vi "MarvinReport.vi"(0 "HEADER1":string="===================================================================\r\n||  Functional and Performance Test  For  DUAL-SERVO- L O W E R  ||\r\n||  P/N  TLM132XX501    S/N:001    Power-Input:18,28,32 +/-0.5V  ||\r\n||  Date:6/12/2007    Time: 15-00  Test-Conductor: Itzik         ||\r\n||  Tester P/N yyyy-yyyyyy-yyyy    S/N:01                        ||\r\n||  POWER SUPPLY P/N xxxxx                                       ||\r\n||  Remarks:                                                     ||\r\n||  You can write here what ever you want                        ||\r\n||                                                               ||\r\n===================================================================", 1 "ATR Or":refnum<vi>, 2 "Steps   pfull":string[][](table)=array602x15[9030 elements] caption="ATR", 3 "Footer UUT":string, 5 "pageNum":i32=13, 6 "InputHeaderArray":string[][](array[string]), 7 "FILE NAME":string="d", 9 "Report Folder":path=path "C:/EPD/ATRS", 11 "PN":string, 12 "error in (no error)":errorcluster, 13 "REV":string, 14 "Test-Conductor":string) -> (4 "path out":path, 15 "error out":errorcluster)   [LabVIEW 2017]
uses:
  <vilib>/Utility/miscctls.llb/LVRowAndColumnUnsignedTypeDef.ctl
  <vilib>/Utility/NIReport.llb/Append Image to Report (path wrap).vi
  <vilib>/Utility/NIReport.llb/Append Text Table to Report (wrap).vi
  <vilib>/Utility/NIReport.llb/Append Report Text (str wrap).vi
  <vilib>/Utility/NIReport.llb/NI_report.lvclass
  <vilib>/Utility/NIReport.llb/Word/NI_Word.lvclass
  <vilib>/addons/_office/NI_ReportGenerationToolkit.lvlib
panel:
  out "Steps   p31":string[][](table)=[["6.1", "Visual Inspection", "", "", "", "", ""], ["6.1.1", "Verification of Components Not Installed", "N/A", "-", "", "", ""], ["", "", "", "", "", "", ""], ["6.1.2", "Manufacturing Defects", "N/A", "-", "", "", ""], ["", "", "", "", "", "", ""], ["6.2", "Power Supply Testing", "", "", "", "", ""], ["6.2.1", "Input Current Drawn", "", "", "", "", ""], ["6.2.1.1", "DC Input Current", "< 150", "-", "mA", "", ""], ["", "", "", "", "", "", ""], ["6.2.2", "Power Supply Voltages", "", "", "", "", ""], ["6.2.2.1", "12V", "12.0", "+/-0.500", "V", "", ""], ["6.2.2.2", "5V", "5.0", "+/-0.200", "V", "", ""], ["6.2.2.3", "3.3V", "3.3", "+/-0.100", "V", "", ""], ["6.2.2.4", "1.8V", "1.8", "+/-0.100", "V", "", ""], ["", "", "", "", "", "", ""], ["7", "Functional Test Procedure", "", "", "", "", ""], ["7.1", "Weight Check", "4180", "+/-10.00", "gr", "", ""], ["", "", "", "", "", "", ""], ["7.2", "Insulation Resistance Test", "", "", "", "", ""], ["7.2.1", "J3.B to Chassis", "> 1M", "-", "ohms", "", ""], ["7.2.2", "J1.16 to Chassis", "> 100K", "-", "ohms", "", ""], ["", "", "", "", "", "", ""], ["7.2", "Bonding Resistance", "", "", "", "", ""], ["7.2.3", "J1 Body to Chassis", "< 2m", "-", "ohms", "", ""], ["7.2.4", "J2  Body to Chassis", "< 2m", "-", "ohms", "", ""], ["7.2.5", "J3  Body to Chassis", "< 2m", "-", "ohms", "", ""], ["", "", "", "", "", "", ""], ["7.2.1", "CANbus Resistance Test", "", "", "", "", ""], ["7.2.1.1", "J1.17 to J1.18", "> 10K", "-", "ohms", "", ""], ["", "", "", "", "", "", ""], ["7.3", "Sealing Test", "N/A", "-", "", "", ""], ["", "", "", "", "", "", ""], ["7.4", "Communication Test", "", "", "", "", ""], ["7.4.1", "Serial RS-232", "N/A", "-", "", "", ""], ["7.4.2", "CAN Bus", "N/A", "-", "", "", ""], ["", "", "", "", "", "", ""], ["7.5", "Performances Tests", "", "", "", "", ""], ["7.5.1", "Reverse Polarity Test", "", "", "", "", ""], ["7.5.1.1", "DC Input Current", "< 1", "-", "mA", "", ""], ["", "", "", "", "", "", ""], ["7.5.2", "Enable Test", "", "", "", "", ""], ["7.5.2.1", "Fan Speed before Opened Enable ", "6000", "+/-200.0", "rpm", "", ""], ["7.5.2.2", "Fan Speed at Opened Enable ", "0", "+/-200.0", "rpm", "", ""], ["7.5.2.3", "Fan Speed at Closed Enable ", "6000", "+/-200.0", "rpm", "", ""], ["7.5.2.4", "Motor Rotation Direction", "Counter-clockwise (Inlet)", "-", "", "", ""], ["", "", "", "", "", "", ""], ["7.5.3", "Stop Time Test ", "", "", "", "", ""], ["7.5.3.1", "Motor Stop time", "< 50", "-", "sec", "", ""], ["", "", "", "", "", "", ""], ["7.5.4", "Speed Command Test", "", "", "", "", ""], ["7.5.4.1", "Fan Speed", "6000", "+/-200.0", "rpm", "", ""], ["7.5.4.2", "Fan Speed", "11500", "+/-200.0", "rpm", "", ""], ["7.5.4.3", "Fan Speed", "15100", "+/-200.0", "rpm", "", ""], ["", "", "", "", "", "", ""], ["7.5.5", "Temperature Sensor Calibration Test", "", "", "", "", ""], ["7.5.5.1", "Sensor Reading Analog Offset", "0", "+/-0.100", ".", "", ""], ["", "", "", "", "", "", ""], ["7.5.6", "Temperature Control Algorithm Test", "", "", "", "", ""], ["7.5.6.1", "Tair <   68 ± 2 oC", "6000", "+/-200.0", "rpm", "", ""], ["7.5.6.2", "Measured Temp.", "", "", "Deg.", "", ""], ["7.5.6.3", "Tair >= 68 ± 2 oC", "11500", "+/-200.0", "rpm", "", ""], ["7.5.6.4", "Transition Temp.", "", "", "Deg.", "", ""], ["7.5.6.5", "Tair >= 88 ± 2 oC", "15100", "+/-400.0", "rpm", "", ""], ["7.5.6.6", "Transition Temp.", "", "", "Deg.", "", ""], ["7.5.6.7", "Tair <= 80 ± 2 oC", "11500", "+/-200.0", "rpm", "", ""], ["7.5.6.8", "Transition Temp.", "", "", "Deg.", "", ""], ["7.5.6.9", "Tair <= 60 ± 2 oC", "6000", "+/-200.0", "rpm", "", ""], ["7.5.6.10", "Transition Temp.", "", "", "Deg.", "", ""], ["", "", "", "", "", "", ""], ["7.5.7", "Burn-in Test", "", "", "", "", ""], ["7.5.7.1", "DC Input Current", "50", "+/-7.000", "A", "", ""], ["7.5.7.2", "Fan Speed", "15100", "+/-400.0", "rpm", "", ""], ["7.5.7.3", "Ambient Temperature", "25", "+/-13.00", "Deg.", "", ""], ["7.5.7.4", "After 10 min of operation", "", "-", "Deg.", "", ""], ["7.5.7.5", "After 20 min of operation", "", "-", "Deg.", "", ""], ["7.5.7.6", "After 30 min of operation", "", "-", "Deg.", "", ""], ["", "", "", "", "", "", ""], ["8", "Auxiliary", "", "", "", "", ""], ["8.1", "Auxiliary Cooling Fan ON", "60", "+/-2.00", "Deg.", "", ""], ["8.2", "Fan status", "ON", "-", "-", "", ""], ["8.3", "Auxiliary Cooling Fan OFF", "55", "+/-2.00", "Deg.", "", ""], ["8.4", "Fan status", "OFF", "-", "-", "", ""], ["", "", "", "", "", "", ""], ["9", "Motor Temp. Test", "", "", "", "", ""], ["9.1", "60 Degree", "60", "+/-2.00", "Deg.", "", ""], ["9.2", "90 Degree", "90", "+/-2.00", "Deg.", "", ""], ["9.3", "110 Degree", "110", "+/-2.00", "Deg.", "", ""]] caption="ATR"
  out "error out 2":errorcluster
  out "RefArr":u32[](array[numeric])
  in  "Tab Control":T1(tab)=enum."Headers and more"
  out "ERRORS\nLIST":string="<pre>Summery of Results (Fails Only) :   Pos.Cmnd.=0.5V F.B. - FAIL !\t   \nPos.Cmnd.=2.0V F.B. - FAIL !\t       Pos.Cmnd.=4.5V F.B. - FAIL !\t  \nPos.Cmnd.=0.5V F.B  - FAIL !\t       Pos.Cmnd.=2.0V F.B. - FAIL !\t\nPos.Cmnd.=4.5V F.B. - FAIL !\t       Pot. / Pos.Cmnd. 1.5v - FAIL !\t   \nPot./Pos.Cmnd.2.0v  - FAIL !\t       Pot. / Pos.Cmnd. 3.5v - FAIL !\t   \nRelay-->RESET  - FAIL !\t            Relay --> SET - FAIL !\t</pre>"
  out "Steps   p1":string[][](table)=[["Load Firmware - reset", "-", "-", "-", "-", ""], ["Test Communication", "-", "-", "-", "-", ""], ["Set S/N", "-", "-", "-", "-", ""], ["Set Board Number", "-", "-", "-", "-", ""], [" ", "", "", "", "", ""], ["Test Communication", "-", "-", "-", "-", ""], ["Get S/N", "-", "-", "-", "", ""], ["Get Board Number", "-", "-", "-", "", ""], ["Get FW", "-", "-", "-", "", ""], ["Small position command", "", "", "", "", ""], ["Measure delta", "", "", "", "", ""], ["Velocity command", "", "", "", "", ""], ["Velocity command", "", "", "", "", ""], ["Velocity command", "", "", "", "", ""], ["Velocity command", "", "", "", "", ""], ["Velocity command", "", "", "", "", ""]] caption="ATR"
  out "Steps   p2":string[][](table)=[["Load Firmware - reset", "-", "-", "-", "-", ""], ["Test Communication", "-", "-", "-", "-", ""], ["Set S/N", "-", "-", "-", "-", ""], ["Set Board Number", "-", "-", "-", "-", ""], [" ", "", "", "", "", ""], ["Test Communication", "-", "-", "-", "-", ""], ["Get S/N", "-", "-", "-", "", ""], ["Get Board Number", "-", "-", "-", "", ""], ["Get FW", "-", "-", "-", "", ""], ["Small position command", "", "", "", "", ""], ["Measure delta", "", "", "", "", ""], ["Velocity command", "", "", "", "", ""], ["Velocity command", "", "", "", "", ""], ["Velocity command", "", "", "", "", ""], ["Velocity command", "", "", "", "", ""], ["Velocity command", "", "", "", "", ""]] caption="ATR"
  out "Steps   p3":string[][](table)=[["Load Firmware - reset", "-", "-", "-", "-", ""], ["Test Communication", "-", "-", "-", "-", ""], ["Set S/N", "-", "-", "-", "-", ""], ["Set Board Number", "-", "-", "-", "-", ""], [" ", "", "", "", "", ""], ["Test Communication", "-", "-", "-", "-", ""], ["Get S/N", "-", "-", "-", "", ""], ["Get Board Number", "-", "-", "-", "", ""], ["Get FW", "-", "-", "-", "", ""], ["Small position command", "", "", "", "", ""], ["Measure delta", "", "", "", "", ""], ["Velocity command", "", "", "", "", ""], ["Velocity command", "", "", "", "", ""], ["Velocity command", "", "", "", "", ""], ["Velocity command", "", "", "", "", ""], ["Velocity command", "", "", "", "", ""]] caption="ATR"
  in  "Fail  Button":bool
  in  "Pass  Button":bool
  # "e"
  # "e"
  # "<pre>"
  # "for html"
  # "for html"
  # "</pre>"
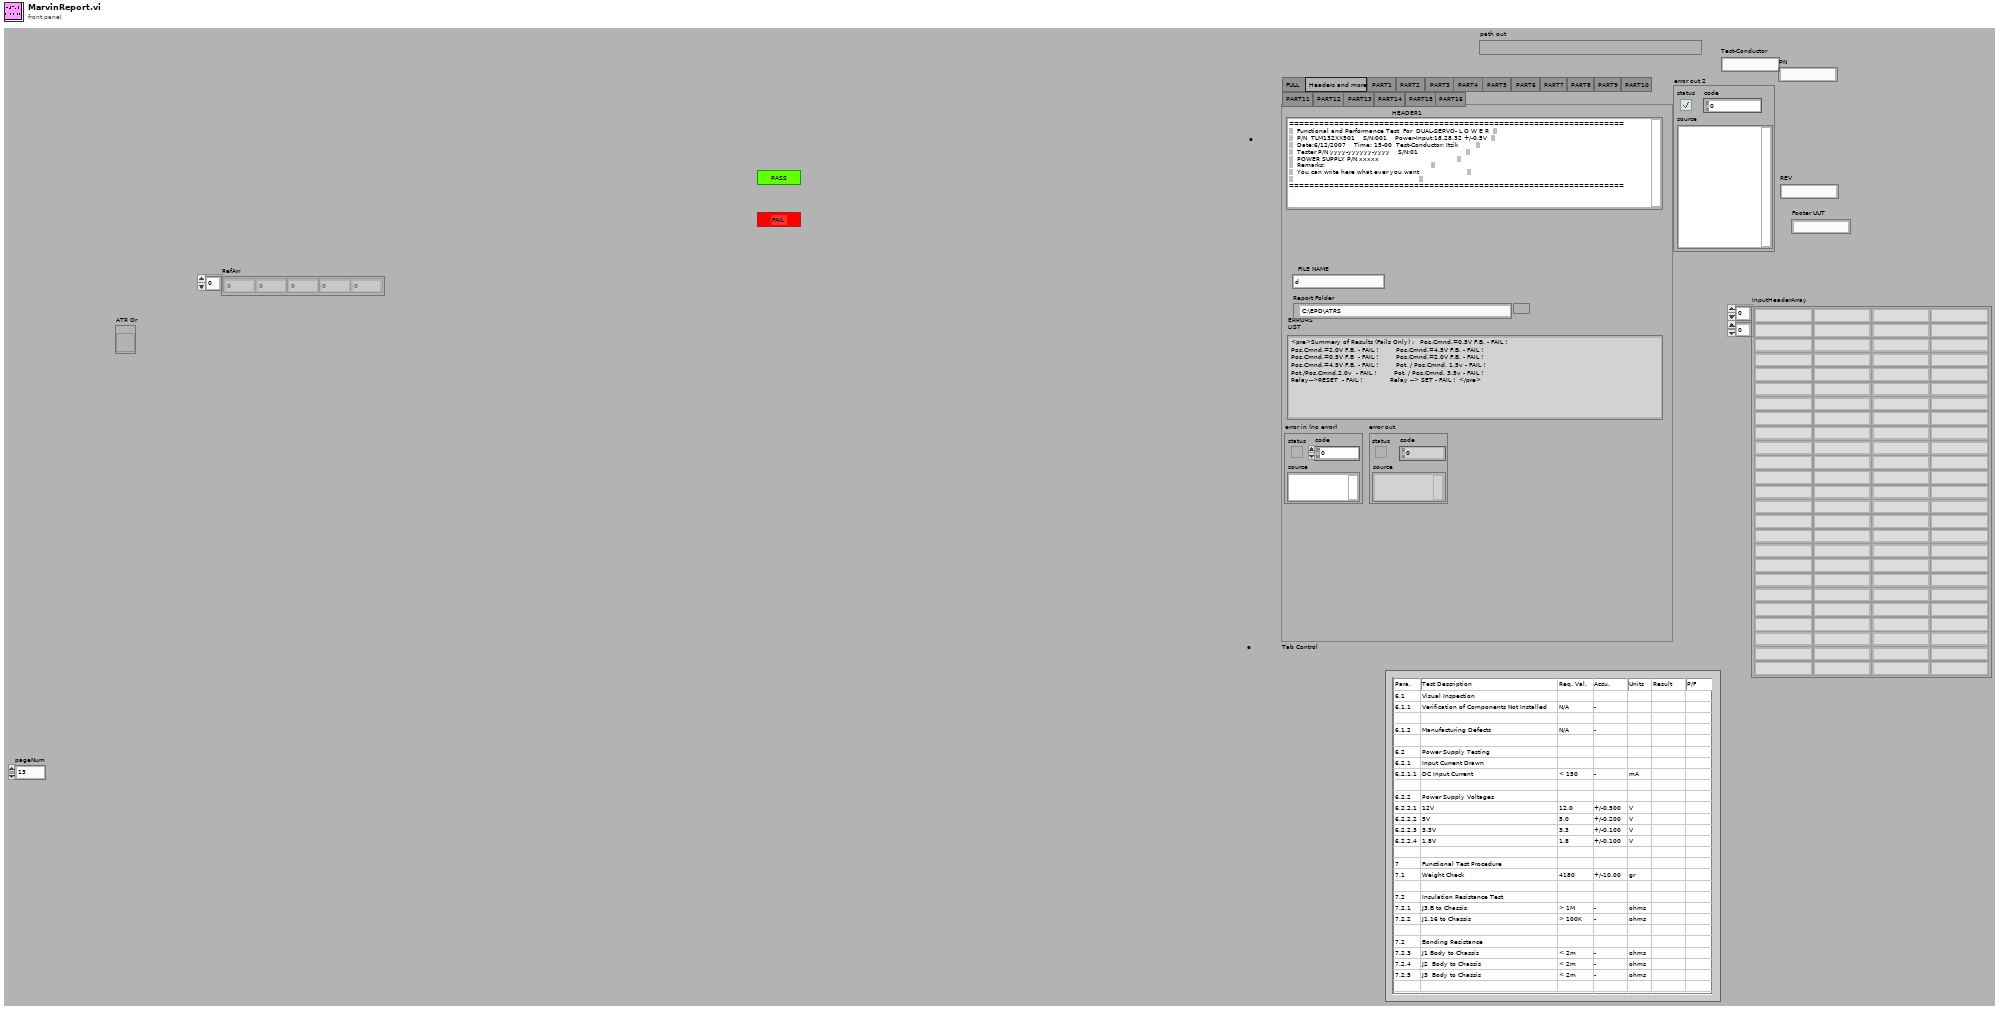
[diagram p1: front panel]
types:
  T1 = enum32{"FULL", "Headers and more", "PART1 ", "PART2 ", "PART3 ", "PART4 ", "PART5 ", "PART6 ", "PART7", "PART8", "PART9", "PART10", "PART11", "PART12", "PART13", "PART14", "PART15", "PART16"}
  T2 = typedef "LVRowAndColumnUnsignedTypeDef.ctl" = cluster{"Row":u32, "Column":u32}
  T3 = cluster{"position (excel)":cluster{"row":i32, "column":i32}, "name (excel)":string, "bookmark (word)":string}
  T4 = cluster{"top":dbl, "left":dbl, "right":dbl, "bottom":dbl}
  T5 = enum16{"Standard Report", "HTML", "Word", "Excel"}
  T6 = cluster{"Italic":enum16{"Italic Unchanged", "Italic On", "Italic Off"}, "Strike Through":enum16{"Strike Through Unchanged", "Strike Through On", "Strike Through Off"}, "Underline":enum16{"Underline Unchanged", "Underline On", "Underline Off"}, "Bold":enum16{"Bold Unchanged", "Bold On", "Bold Off"}}
  T7 = cluster{"charset (-1)":i16, "weight (-1)":i16, "name":string, "size":string}
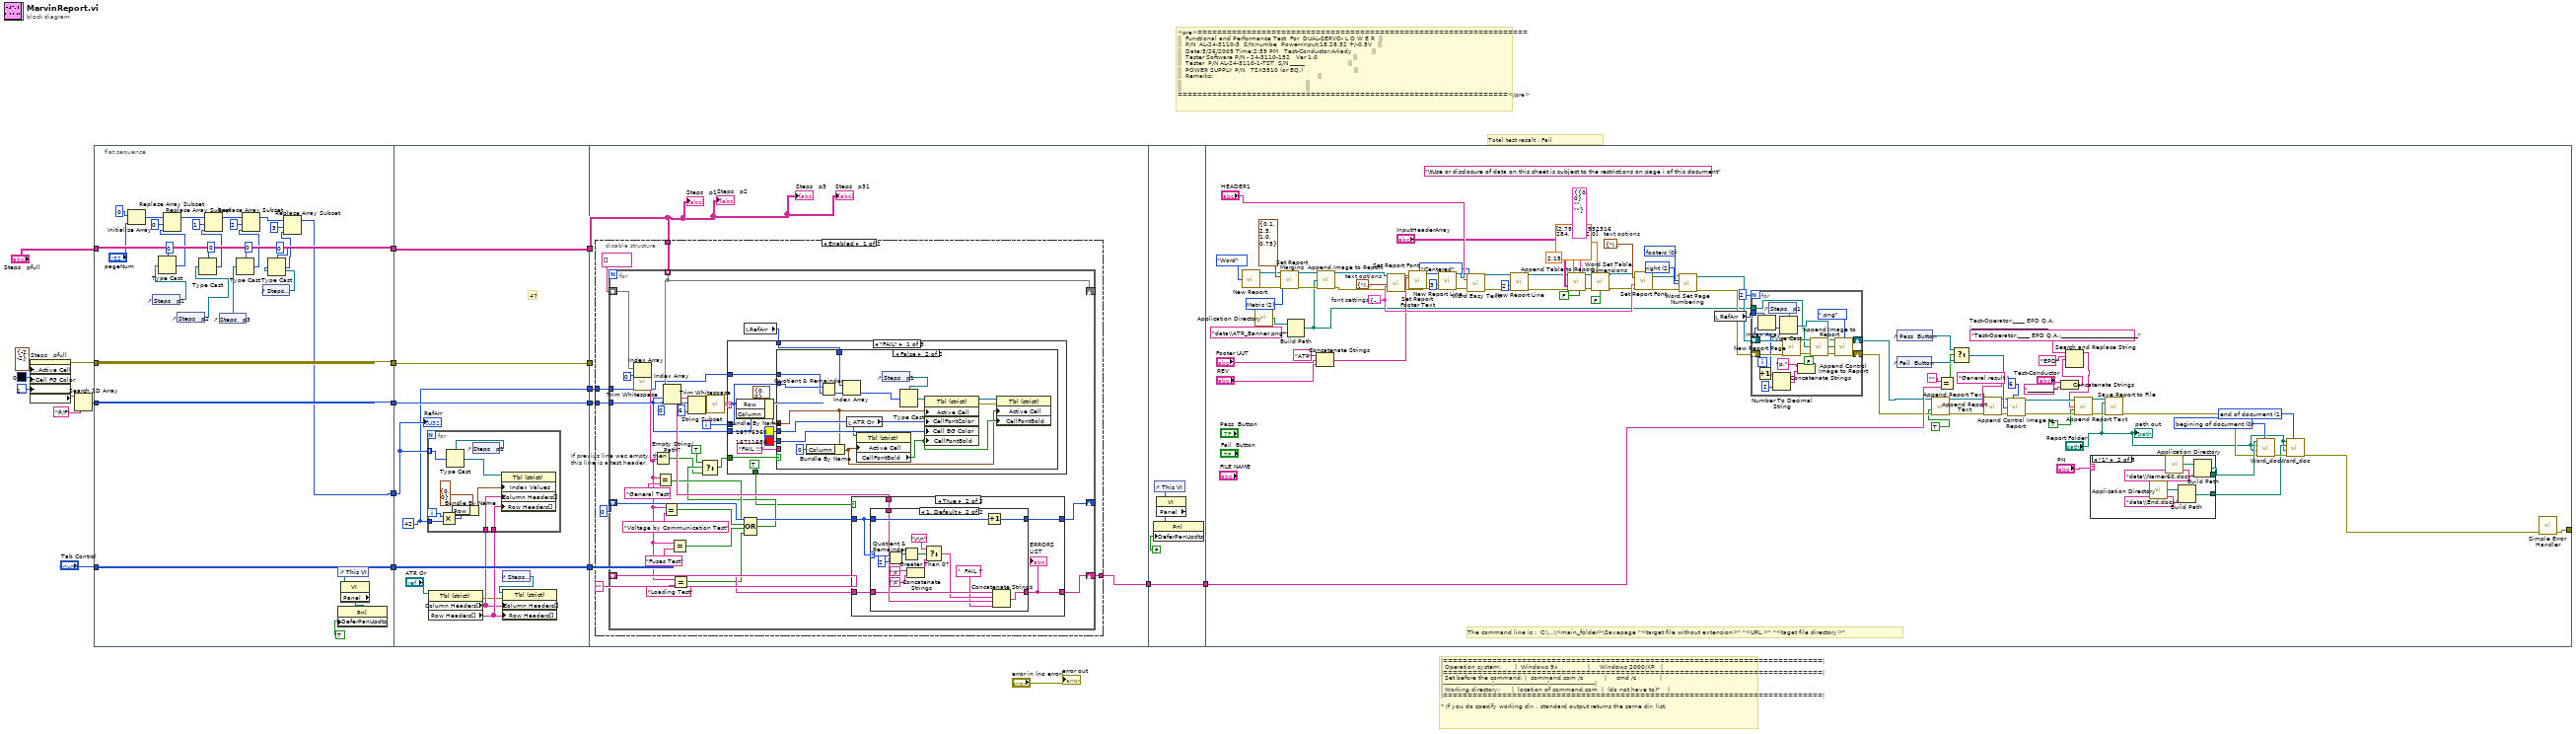
[diagram p0: block diagram]
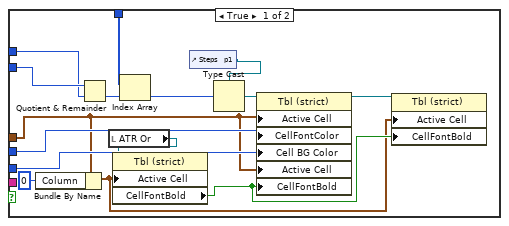
[diagram p2: hidden frame]
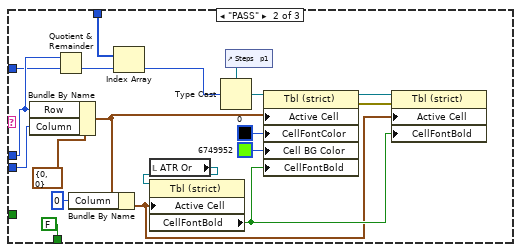
[diagram p3: hidden frame]
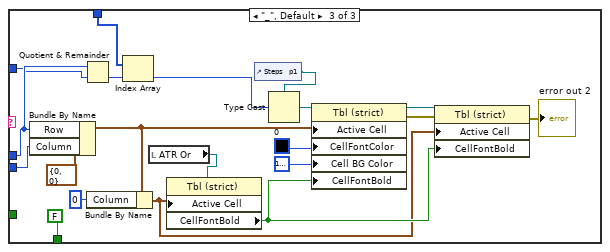
[diagram p4: hidden frame]
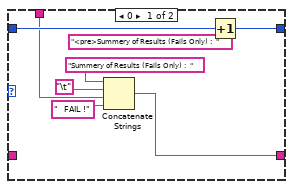
[diagram p6: hidden frame]
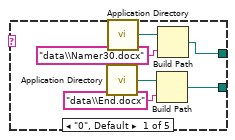
[diagram p8: hidden frame]
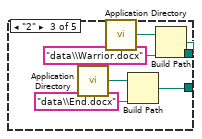
[diagram p9: hidden frame]
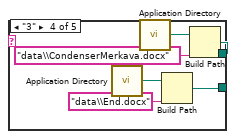
[diagram p10: hidden frame]
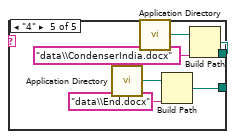
[diagram p11: hidden frame]
diagram:
  # "Total test resalt : Fail"
  # "|=============================================================================|\n| Operation system:       |  Windows 9x               |     Windows 2000/XP   |\n|=============================================================================|\n| Set before the command: |  command.com /c           |     cmd /c            |\n|-------------------------|---------------------------|-----------------------|\n| Working directory:      |  location of command.com  |  (do not have to)*    |\n|=============================================================================|\n\n* If you do specify working dir. , standard output returns the same dir. list."
  # "<pre>===================================================================\n||  Functional and Performance Test  For  DUAL-SERVO- L O W E R  ||\n||  P/N  AL-24-3110-3  S/N:numbe  Power-Input:18,28,32 +/-0.5V   ||\n||  Date:5/26/2005 Time:2:59 PM   Test-Conductor:Arkady          ||\n||  Tester Software P/N - 24-3110-152   Ver 1.0                  ||\n||  Tester  P/N AL-24-3110-1-TST  S/N _____                      ||\n||  POWER SUPPLY P/N   TSX3510 (or EQ.)                          ||\n||  Remarks:                                                     ||\n||                                                               ||\n||                                                               ||\n===================================================================</pre>"
  n1 = property on="Steps   pfull" class="Tbl (strict)"("Active Cell:Active Cell"=cluster{"Row":i32, "Column":i32} {"Row"=-2, "Column"=-2} ("Active Cell"), "Active Cell:Cell FG Color"=u32 0, "Active Cell:Cell Background Color"=u32 16777226) -> (error out=w19:errorcluster, "Column Header Strings[]"=w17:string[])  [unwired: 2 in, 1 out]
  n2 = Search 1D Array(1D array=w17, element="P/F") -> (index of element=w16:i32)  [unwired: 1 in]
  n3 = flat-sequence {
    tunnel: "Tab Control" -> [w49]
    tunnel: w16 -> [w50]
    tunnel: w19 -> [w51]
    tunnel: "Steps   pfull" -> [w52]
    tunnel: [w52] -> w8
    tunnel: [w51] -> w7
    tunnel: [w50] -> w6
    tunnel: [w49] -> w5
    tunnel: [w27] -> w2
    tunnel: [w63] -> w12
    tunnel: [w62] -> w11
    tunnel: [w61] -> w10
    tunnel: [w60] -> w9
    tunnel: w8 -> [w63]
    tunnel: w7 -> [w62]
    tunnel: w6 -> [w61]
    tunnel: w5 -> [w60]
    tunnel: w2 -> [w55]
    tunnel: [w53] -> w1
    tunnel: [w76] -> w4
    tunnel: w12 -> [w74]
    tunnel: w11 -> [_]
    tunnel: w10 -> [w77]
    tunnel: w9 -> [_]
    tunnel: w1 -> [w75]
    tunnel: w4 -> [w230]
    tunnel: [w230] -> w3
    tunnel: [w316] -> _
    tunnel: w3 -> [w303]
    frame #0 {
      n4 = Initialize Array "Initialize Array"(u32 0, "pageNum") -> (w34:u32[])
      n5 = control-ref of="Steps   p1"() -> (w45:refnum<vi>)
      n6 = Type Cast(type=u32 0, x=w45) -> (*(type *) &x=w35:u32)
      n7 = Replace Array Subset(array=w34, new element=w35, index=0) -> (w38:u32[])
      n8 = control-ref of="Steps   p2"() -> (w30:refnum<vi>)
      n9 = Type Cast(type=u32 0, x=w30) -> (*(type *) &x=w39:u32)
      n10 = Replace Array Subset(array=w38, new element=w39, index=1) -> (w44:u32[])
      n11 = control-ref of="Steps   p3"() -> (w24:refnum<vi>)
      n12 = Type Cast(type=u32 0, x=w24) -> (*(type *) &x=w42:u32)
      n13 = Replace Array Subset(array=w44, new element=w42, index=2) -> (w28:u32[])
      n14 = control-ref of="Steps   p31"() -> (w23:refnum<vi>)
      n15 = Type Cast(type=u32 0, x=w23) -> (*(type *) &x=w25:u32)
      n16 = Replace Array Subset(array=w28, new element=w25, index=3) -> (w27:u32[])
      n17 = control-ref of="This VI"() -> (w46:refnum<vi>)
      n18 = property class="VI"(reference=w46) -> ("Panel"=w47:refnum<vi>)  [unwired: 1 in, 2 out]
      n19 = property class="Pnl"(reference=w47, "DeferPanUpdts"=TRUE ("Defer Panel Updates")) -> ()  [unwired: 1 in, 2 out]
    }
    frame #1 {
      w53 = u32 42 ("Row")
      # "47"
      n20 = property class="Tbl (strict)"(reference="ATR Or") -> (error out=w57:errorcluster, "Column Headers[]"=w58:string[], "Row Headers[]"=w59:string[])  [unwired: 1 in, 1 out]
      n21 = for {
        tunnel: w55 -> [w73] mode=indexing
        tunnel: w58 -> [w67]
        tunnel: w59 -> [w66]
        tunnel: w53 -> [w64]
        i -> [w69]
        n22 = Multiply(x=w69, y=w64) -> (x*y=w68:u32)
        n23 = Bundle By Name(cluster=T2 {"Row"=0, "Column"=0} ("Index Values"), "Row"=w68) -> (w70:T2)
        n24 = control-ref of="Steps   p1"() -> (w65:refnum<vi>)
        n25 = Type Cast(type=w65, x=w73) -> (*(type *) &x=w72:refnum<vi>)
        n26 = property class="Tbl (strict)"(reference=w72, "Index Values"=w70, "Column Headers[]"=w67, "Row Headers[]"=w66) -> ()  [unwired: 1 in, 2 out]
      }
      n27 = control-ref of="Steps   pfull"() -> (w54:refnum<vi>)
      n28 = property class="Tbl (strict)"(reference=w54, error in=w57, "Column Headers[]"=w58, "Row Headers[]"=w59) -> ()  [unwired: 2 out]
      "RefArr" <- w55
    }
    frame #2 {
      n29 = disable-structure shown="Enabled" {
        disable-tunnel: w77 -> [w84 _]
        disable-tunnel: [w83 _] -> w76
        disable-tunnel: w74 -> [w79 _]
        disable-tunnel: w75 -> [w78 _]
        frame Enabled {
          n30 = for {
            tunnel: w79 -> [w114] mode=indexing
            shift-right: [w114] -> _
            shift-left: string[] [] ("ATR in") -> [w113]
            tunnel: w84 -> [w90]
            shift-right: [w105] -> w83
            shift-left: "" ("trimmed string") -> [w109]
            shift-right: [w108] -> _
            shift-left: 0 -> [w107]
            tunnel: w78 -> [w85]
            i -> [w91]
            n31 = Index Array(array=w113, index=0) -> (element=w111:string)
            n32 = call <vilib>:"Trim Whitespace.vi"("string"=w111) -> ("trimmed string"=w86:string)  [unwired: 1 in]
            n33 = Empty String/Path? "If previus line was empty, then\nthis line is a test header."(string/path=w86) -> (empty?=w93:bool)
            n34 = Equal?(x=w86, y="General Test") -> (x = y?=w102:bool)
            n35 = Equal?(x=w86, y="Voltage by Communication Test") -> (x = y?=w97:bool)
            n36 = Index Array(array=w114, index #1=w90, index #2=0) -> (element #1=w110:string, element #2=w106:string)
            n37 = Equal?(x=w86, y="Fuses Test") -> (x = y?=w98:bool)
            n38 = Equal?(x=w86, y="Loading Test") -> (x = y?=w99:bool)
            n39 = String Subset(string=w110, length (rest)=6 ("length (rest)")) -> (substring=w115:string)  [unwired: 1 in]
            n40 = call <vilib>:"Trim Whitespace.vi"("string"=w115) -> ("trimmed string"=w92:string)  [unwired: 1 in]
            n41 = local read "RefArr"() -> (w87:u32[])
            n42 = Compound Arithmetic op=OR(w102, w97, w98, w99) -> (w100:bool)
            n43 = Select(t=TRUE, s=w100, f=w93) -> (s? t:f=w89:bool)
            n44 = case shown="\"FAIL\"" w92 {
              tunnel: w91 -> [w119 w172 w193]
              tunnel: w90 -> [w121 w176 w196]
              tunnel: w89 -> [w123 _ _]
              tunnel: [TRUE FALSE FALSE] -> w88
              tunnel: w87 -> [w120 w170 w192]
              tunnel: w85 -> [w117 w159 w178]
              frame "FAIL" {
                n45 = Bundle By Name(cluster=cluster{"Row":i32, "Column":i32} {"Row"=0, "Column"=0} ("Active Cell"), "Row"=w119, "Column"=w121) -> (w127:cluster{"Row":i32, "Column":i32})
                n46 = case shown="False" w123 {
                  tunnel: w127 -> [w135 w147]
                  tunnel: u32 16776960 -> [w142 w158]
                  tunnel: u32 16711680 -> [w141 w157]
                  tunnel: "FAIL !!!" ("string") -> [_ _]
                  tunnel: w120 -> [w139 w154]
                  tunnel: w119 -> [w138 w155]
                  tunnel: w117 -> [w128 w143]
                  frame True {
                    n47 = Bundle By Name(cluster=w135, "Column"=0) -> (w131:cluster{"Row":i32, "Column":i32})
                    n48 = Quotient & Remainder(x=w138, y=w128) -> (floor(x/y)=w140:u32)  [unwired: 1 out]
                    n49 = local read "ATR Or"() -> (w129:refnum<vi>)
                    n50 = property class="Tbl (strict)"(reference=w129, "Active Cell"=w131) -> ("CellFontBold"=w132:bool)  [unwired: 1 in, 2 out]
                    n51 = Index Array(array=w139, index=w140) -> (element=w136:u32)
                    n52 = control-ref of="Steps   p1"() -> (w130:refnum<vi>)
                    n53 = Type Cast(type=w130, x=w136) -> (*(type *) &x=w137:refnum<vi>)
                    n54 = property class="Tbl (strict)"(reference=w137, "Active Cell"=w135, "CellFontColor"=w142, "Cell BG Color"=w141, "Active Cell"=w135, "CellFontBold"=w132) -> (reference out=w133:refnum<vi>)  [unwired: 1 in, 1 out]
                    n55 = property class="Tbl (strict)"(reference=w133, "Active Cell"=w131, "CellFontBold"=w132) -> ()  [unwired: 1 in, 2 out]
                  }
                  frame False {
                    n56 = Bundle By Name(cluster=w147, "Column"=0) -> (w146:cluster{"Row":i32, "Column":i32})
                    n57 = Quotient & Remainder(x=w155, y=w143) -> (floor(x/y)=w156:u32)  [unwired: 1 out]
                    n58 = Index Array(array=w154, index=w156) -> (element=w153:u32)
                    n59 = local read "ATR Or"() -> (w145:refnum<vi>)
                    n60 = property class="Tbl (strict)"(reference=w145, "Active Cell"=w146) -> ("CellFontBold"=w149:bool)  [unwired: 1 in, 2 out]
                    n61 = control-ref of="Steps   p1"() -> (w144:refnum<vi>)
                    n62 = Type Cast(type=w144, x=w153) -> (*(type *) &x=w152:refnum<vi>)
                    n63 = property class="Tbl (strict)"(reference=w152, "Active Cell"=w147, "CellFontColor"=w158, "Cell BG Color"=w157, "CellFontBold"=w149) -> (reference out=w151:refnum<vi>, error out=w150:errorcluster)  [unwired: 1 in]
                    n64 = property class="Tbl (strict)"(reference=w151, error in=w150, "Active Cell"=w146, "CellFontBold"=w149) -> ()  [unwired: 2 out]
                  }
                }
              }
              frame "PASS" {
                n65 = Bundle By Name(cluster=cluster{"Row":i32, "Column":i32} {"Row"=0, "Column"=0} ("Active Cell"), "Row"=w172, "Column"=w176) -> (w163:cluster{"Row":i32, "Column":i32})
                n66 = Quotient & Remainder(x=w172, y=w159) -> (floor(x/y)=w171:u32)  [unwired: 1 out]
                n67 = Bundle By Name(cluster=w163, "Column"=0) -> (w162:cluster{"Row":i32, "Column":i32})
                n68 = Index Array(array=w170, index=w171) -> (element=w169:u32)
                n69 = local read "ATR Or"() -> (w160:refnum<vi>)
                n70 = property class="Tbl (strict)"(reference=w160, "Active Cell"=w162) -> ("CellFontBold"=w165:bool)  [unwired: 1 in, 2 out]
                n71 = control-ref of="Steps   p1"() -> (w161:refnum<vi>)
                n72 = Type Cast(type=w161, x=w169) -> (*(type *) &x=w168:refnum<vi>)
                n73 = property class="Tbl (strict)"(reference=w168, "Active Cell"=w163, "CellFontColor"=u32 0, "Cell BG Color"=u32 6749952, "CellFontBold"=w165) -> (reference out=w166:refnum<vi>, error out=w167:errorcluster)  [unwired: 1 in]
                n74 = property class="Tbl (strict)"(reference=w166, error in=w167, "Active Cell"=w162, "CellFontBold"=w165) -> ()  [unwired: 2 out]
              }
              frame "_", Default {
                n75 = Bundle By Name(cluster=cluster{"Row":i32, "Column":i32} {"Row"=0, "Column"=0} ("Active Cell"), "Row"=w193, "Column"=w196) -> (w186:cluster{"Row":i32, "Column":i32})
                n76 = Quotient & Remainder(x=w193, y=w178) -> (floor(x/y)=w194:u32)  [unwired: 1 out]
                n77 = Bundle By Name(cluster=w186, "Column"=0) -> (w182:cluster{"Row":i32, "Column":i32})
                n78 = Index Array(array=w192, index=w194) -> (element=w191:u32)
                n79 = local read "ATR Or"() -> (w180:refnum<vi>)
                n80 = property class="Tbl (strict)"(reference=w180, "Active Cell"=w182) -> ("CellFontBold"=w183:bool)  [unwired: 1 in, 2 out]
                n81 = control-ref of="Steps   p1"() -> (w181:refnum<vi>)
                n82 = Type Cast(type=w181, x=w191) -> (*(type *) &x=w188:refnum<vi>)
                n83 = property class="Tbl (strict)"(reference=w188, "Active Cell"=w186, "CellFontColor"=u32 0, "Cell BG Color"=u32 16777226, "CellFontBold"=w183) -> (reference out=w185:refnum<vi>, error out=w184:errorcluster)  [unwired: 1 in]
                n84 = property class="Tbl (strict)"(reference=w185, error in=w184, "Active Cell"=w182, "CellFontBold"=w183) -> (error out=→"error out 2":errorcluster)  [unwired: 1 out]
              }
            }
            n85 = case shown="True" w88 {
              tunnel: w109 -> [w199 w201]
              tunnel: [w199 w200] -> w105
              tunnel: w107 -> [w198 w203]
              tunnel: [w198 w204] -> w108
              tunnel: w106 -> [_ w202]
              frame False {
              }
              frame True {
                n86 = case shown="1, Default" w203 {
                  selector: w203 -> [_ w225]
                  tunnel: [w206 w215] -> w204
                  tunnel: w203 -> [w211 w226]
                  tunnel: w202 -> [w210 w222]
                  tunnel: [w208 w221] -> w200
                  tunnel: w201 -> [_ w220]
                  frame 0 {
                    (unwired) "<pre>Summery of Results (Fails Only) :  "
                    n87 = Concatenate Strings("Summery of Results (Fails Only) :  ", "\t", w210, "  FAIL !" ("string")) -> (w208:string)
                    n88 = Increment(x=w211) -> (x+1=w206:i32)
                  }
                  frame 1, Default {
                    n89 = Quotient & Remainder(x=w225, y=2) -> (x-y*floor(x/y)=w223:i32)  [unwired: 1 out]
                    n90 = Greater Than 0?(x=w223) -> (x > 0?=w219:bool)
                    n91 = Concatenate Strings("\t", "\t") -> (w214:string)
                    n92 = Select(t="\r\n", s=w219, f=w214) -> (s? t:f=w217:string)
                    n93 = Increment(x=w226) -> (x+1=w215:i32)
                    n94 = Concatenate Strings(w220, w217, w222, "  FAIL !" ("string")) -> (w221:string)
                  }
                }
                "ERRORS\nLIST" <- w200
              }
            }
          }
        }
        frame Disabled {
        }
      }
      "Steps   p1" <- w74
      "Steps   p2" <- w74
      "Steps   p31" <- w74
      "Steps   p3" <- w74
    }
    frame #3 {
      n95 = control-ref of="This VI"() -> (w227:refnum<vi>)
      n96 = property class="VI"(reference=w227) -> ("Panel"=w228:refnum<vi>)  [unwired: 1 in, 2 out]
      n97 = property class="Pnl"(reference=w228, "DeferPanUpdts"=FALSE ("Defer Panel Updates")) -> ()  [unwired: 1 in, 2 out]
    }
    frame #4 {
      w232 = u16 1 items=["begining of document", "end of document", "bookmark", "Custom"] ("insertion point")
      w236 = u16 0 items=["begining of document", "end of document", "bookmark", "Custom"] ("insertion point")
      w274 = u16 2 items=["Default", "US", "Metric"] ("measurement system (default)")
      (unwired) "\tUse or disclosure of data on this sheet is subject to the restrictions on page i of this document" ("center footer text")
      w283 = u16 2 items=["left", "center", "right"] ("alignment (right)")
      w284 = u16 0 items=["footers", "headers"] ("position (footers)")
      w304 = T6 {"Italic"=enum."Italic Off", "Strike Through"=enum."Strike Through Off", "Underline"=enum."Underline Off", "Bold"=enum."Bold Off"}  # text options
      w317 = T6 {"Italic"=enum."Italic Off", "Strike Through"=enum."Strike Through Off", "Underline"=enum."Underline Off", "Bold"=enum."Bold Off"}  # text options
      w301 = "Test-Operator:____ EPD Q.A.:__________________________"  # Test-Operator:____ EPD Q.A.:__________________________
      w305 = T7 {"charset (-1)"=-1, "weight (-1)"=-1, "name"="Tahoma", "size"="12"}  # font settings
      # "The command line is :  C:\\...\\<main_folder>\\Savepage \"<target file without extension>\" \"<URL >\" \"<taget file directory>\""
      n98 = call <vilib>:"New Report.vi"("report type"=T5."Word") -> ("report out"=w272:refnum<class "NI_report.lvclass">, "error out"=w273:errorcluster)  [unwired: 13 in]
      n99 = call <vilib>:"Application Directory.vi"() -> ("Application Directory"=w267:path)
      n100 = call-dynamic "Set Report Margins.vi"("report in"=w272, "margins (1.00)"=T4 {"top"=0.1, "left"=2.5, "right"=1.0, "bottom"=0.75}, "measurement system (default)"=w274, "error in (no error)"=w273) -> ("report out"=w271:refnum<class "NI_report.lvclass">, "error out"=w270:errorcluster)  [unwired: 9 in, 1 out]
      n101 = Build Path(base path=w267, name or relative path="data\\ATR_Banner.png") -> (appended path=w265:path)
      n102 = Concatenate Strings("ATR" ("string"), "Footer UUT", "REV") -> (w277:string)
      n103 = call-poly <vilib>:"Append Image to Report.vi"("report in"=w271, "path or URL of image"=w265, "error in (no error)"=w270) -> ("report out"=w268:refnum<class "NI_report.lvclass">, "error out"=w269:errorcluster)  [unwired: 9 in, 2 out]
      n104 = call-dynamic "Set Report Font.vi"("report in"=w268, "text options"=w317, "font settings"=w305, "error in (no error)"=w269) -> ("report out"=w292:refnum<class "NI_report.lvclass">, "error out"=w289:errorcluster)  [unwired: 9 in, 1 out]
      n105 = call-dynamic "Set Report Footer Text.vi"("report in"=w292, "left footer text"=w277, "error in (no error)"=w289) -> ("report out"=w291:refnum<class "NI_report.lvclass">, "error out"=w290:errorcluster)  [unwired: 11 in]
      n106 = call-dynamic "New Report Line.vi"("report in"=w291, "number of lines (1)"=3, "error in (no error)"=w290) -> ("report out"=w258:refnum<class "NI_report.lvclass">, "error out"=w257:errorcluster)  [unwired: 11 in]
      n107 = call <vilib>:"Word Easy Text.vi"("report in"=w258, "text"="HEADER1", "alignment (left)"=enum16{"Left", "Centered", "Right", "Justify"}."Centered", "error in (no error)"=w257) -> ("report out"=w243:refnum<class "NI_report.lvclass">, "error out"=w244:errorcluster)  [unwired: 9 in, 1 out]
      n108 = call-dynamic "New Report Line.vi"("report in"=w243, "number of lines (1)"=2, "error in (no error)"=w244) -> ("report out"=w242:refnum<class "NI_report.lvclass">, "error out"=w241:errorcluster)  [unwired: 11 in]
      n109 = call-poly <vilib>:"Append Table to Report.vi"("report in"=w242, "column width (1)"=2.15, "MS Office parameters"=T3 {"position (excel)"={"row"=0, "column"=0}, "name (excel)"="", "bookmark (word)"=""}, "text data"="InputHeaderArray", "error in (no error)"=w241, "show grid lines (YES)"=FALSE) -> ("report out"=w249:refnum<class "NI_report.lvclass">, "error out"=w248:errorcluster)  [unwired: 6 in, 2 out]
      n110 = call <vilib>:"Word Set Table Dimensions.vi"("report in"=w249, "table column widths"=sgl[] [2.8, 2.0, 2.0], "error in (no error)"=w248, "fit to page width? (F)"=FALSE) -> ("report out"=w251:refnum<class "NI_report.lvclass">, "error out"=w252:errorcluster)  [unwired: 10 in]
      n111 = call-dynamic "Set Report Font.vi"("report in"=w251, "text options"=w304, "font settings"=w305, "error in (no error)"=w252) -> ("report out"=w262:refnum<class "NI_report.lvclass">, "error out"=w261:errorcluster)  [unwired: 9 in, 1 out]
      n112 = call <vilib>:"Word Set Page Numbering.vi"("report in"=w262, "position (footers)"=w284, "alignment (right)"=w283, "error in (no error)"=w261) -> ("report out"=w286:refnum<class "NI_report.lvclass">, "error out"=w285:errorcluster)  [unwired: 10 in]
      n113 = local read "RefArr"() -> (w281:u32[])
      n114 = for {
        N: 2 -> [_]
        tunnel: w281 -> [w355]
        shift-right: [w360] -> w288
        shift-left: w285 -> [w361]
        shift-right: [w359] -> w287
        shift-left: w286 -> [w362]
        tunnel: w265 -> [w348]
        i -> [w353]
        (unwired) FALSE ("append on new line? (F)")
        n115 = Increment(x=w353) -> (x+1=w365:i32)
        n116 = Index Array(array=w355, index=w353) -> (element=w354:u32)
        n117 = control-ref of="Steps   p1"() -> (w357:refnum<vi>)
        n118 = Number To Decimal String(number=w365, width (-)=i16 2) -> (decimal integer string=w363:string)
        n119 = Type Cast(type=w357, x=w354) -> (*(type *) &x=w358:refnum<vi>)
        n120 = call-dynamic "New Report Page.vi"("report in"=w362, "error in (no error)"=w361) -> ("report out"=w351:refnum<class "NI_report.lvclass">, "error out"=w352:errorcluster)  [unwired: 12 in]
        n121 = Concatenate Strings("p.", w363) -> ()  [unwired: 1 out]
        n122 = call-poly <vilib>:"Append Image to Report.vi"("report in"=w351, "path or URL of image"=w348, "error in (no error)"=w352) -> ("report out"=w350:refnum<class "NI_report.lvclass">, "error out"=w349:errorcluster)  [unwired: 9 in, 2 out]
        n123 = call-dynamic "Append Control Image to Report.vi"("report in"=w350, "image file type (.jpg)"=enum16{".jpg", ".png"}.".png" ("image file type(.jpg)"), "ctrl reference"=w358, "error in (no error)"=w349) -> ("report out"=w359:refnum<class "NI_report.lvclass">, "error out"=w360:errorcluster)  [unwired: 8 in, 2 out]
      }
      n124 = control-ref of="Fail  Button"() -> (w312:refnum<vi>)
      n125 = control-ref of="Pass  Button"() -> (w313:refnum<vi>)
      n126 = call-poly <vilib>:"Append Report Text.vi"("report in"=w287, "append on new line? (F)"=TRUE, "error in (no error)"=w288) -> ("report out"=w260:refnum<class "NI_report.lvclass">, "error out"=w259:errorcluster)  [unwired: 9 in, 2 out]
      n127 = Equal?(x="", y=w303) -> (x = y?=w310:bool)
      n128 = Select(t=w313, s=w310, f=w312) -> (s? t:f=w314:refnum<vi>)
      n129 = call-poly <vilib>:"Append Report Text.vi"("report in"=w260, "text"="General result:", "error in (no error)"=w259) -> ("report out"=w308:refnum<class "NI_report.lvclass">, "error out"=w309:errorcluster)  [unwired: 9 in, 2 out]
      n130 = call-dynamic "Append Control Image to Report.vi"("report in"=w308, "alignment (default)"=6, "ctrl reference"=w314, "error in (no error)"=w309) -> ("report out"=w306:refnum<class "NI_report.lvclass">, "error out"=w307:errorcluster)  [unwired: 8 in, 2 out]
      n131 = Concatenate Strings("Test-Conductor", "_________") -> (w296:string)
      n132 = Search and Replace String(input string=w301, search string="EPD", replace string=w296) -> (result string=w298:string)  [unwired: 5 in, 3 out]
      n133 = call-poly <vilib>:"Append Report Text.vi"("report in"=w306, "text"=w298, "append on new line? (F)"=TRUE, "error in (no error)"=w307) -> ("report out"=w294:refnum<class "NI_report.lvclass">, "error out"=w293:errorcluster)  [unwired: 8 in, 2 out]
      n134 = case shown="\"1\"" "PN" {
        tunnel: [w321 w327 w333 w339 w345] -> w238
        tunnel: [w318 w324 w330 w336 w342] -> w234
        frame "0", Default {
          n135 = call <vilib>:"Application Directory.vi"() -> ("Application Directory"=w319:path)
          n136 = call <vilib>:"Application Directory.vi"() -> ("Application Directory"=w323:path)
          n137 = Build Path(base path=w319, name or relative path="data\\End.docx") -> (appended path=w318:path)
          n138 = Build Path(base path=w323, name or relative path="data\\Namer30.docx") -> (appended path=w321:path)
        }
        frame "1" {
          n139 = call <vilib>:"Application Directory.vi"() -> ("Application Directory"=w325:path)
          n140 = call <vilib>:"Application Directory.vi"() -> ("Application Directory"=w329:path)
          n141 = Build Path(base path=w325, name or relative path="data\\End.docx") -> (appended path=w324:path)
          n142 = Build Path(base path=w329, name or relative path="data\\Namer60.docx") -> (appended path=w327:path)
        }
        frame "2" {
          n143 = call <vilib>:"Application Directory.vi"() -> ("Application Directory"=w331:path)
          n144 = call <vilib>:"Application Directory.vi"() -> ("Application Directory"=w335:path)
          n145 = Build Path(base path=w331, name or relative path="data\\End.docx") -> (appended path=w330:path)
          n146 = Build Path(base path=w335, name or relative path="data\\Warrior.docx") -> (appended path=w333:path)
        }
        frame "3" {
          n147 = call <vilib>:"Application Directory.vi"() -> ("Application Directory"=w337:path)
          n148 = call <vilib>:"Application Directory.vi"() -> ("Application Directory"=w341:path)
          n149 = Build Path(base path=w337, name or relative path="data\\End.docx") -> (appended path=w336:path)
          n150 = Build Path(base path=w341, name or relative path="data\\CondenserMerkava.docx") -> (appended path=w339:path)
        }
        frame "4" {
          n151 = call <vilib>:"Application Directory.vi"() -> ("Application Directory"=w343:path)
          n152 = call <vilib>:"Application Directory.vi"() -> ("Application Directory"=w347:path)
          n153 = Build Path(base path=w343, name or relative path="data\\End.docx") -> (appended path=w342:path)
          n154 = Build Path(base path=w347, name or relative path="data\\CondenserIndia.docx") -> (appended path=w345:path)
        }
      }
      n155 = call-dynamic "Save Report to File.vi"("report in"=w294, "report file path"="Report Folder", "error in (no error)"=w293) -> ("error out"=w237:errorcluster)  [unwired: 11 in, 1 out]
      n156 = call "Word_doc.vi"("insertion point"=w236, "error in (no error)"=w237, "report file path out"="Report Folder", "Report in 2"="Report Folder", "Report in 1"=w238) -> ("error out"=w235:errorcluster)  [unwired: 6 in]
      n157 = call "Word_doc.vi"("insertion point"=w232, "error in (no error)"=w235, "report file path out"="Report Folder", "Report in 2"=w234, "Report in 1"="Report Folder") -> ("error out"=w231:errorcluster)  [unwired: 6 in]
      n158 = call <vilib>:"Simple Error Handler.vi"("error in (no error)"=w231) -> ("error out"=w316:errorcluster)  [unwired: 4 in, 4 out]
      "path out" <- "Report Folder"
    }
  }
  "error out" <- "error in (no error)"
